vi "operators.vi"() -> ()   [LabVIEW 2019]
panel:
  out "a/b":dbl
  out "axb":dbl
  out "a-b":dbl
  out "a+b":dbl
  in  "b":dbl
  in  "a":dbl
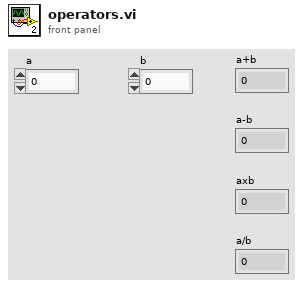
[diagram p1: front panel]
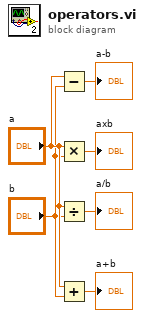
[diagram p0: block diagram]
diagram:
  n1 = Subtract(x="a", y="b") -> (x-y=→"a-b":dbl)
  n2 = Multiply(x="a", y="b") -> (x*y=→"axb":dbl)
  n3 = Divide(x="a", y="b") -> (x/y=→"a/b":dbl)
  n4 = Add(x="a", y="b") -> (x+y=→"a+b":dbl)
